vi "SaveConfigFile.vi"(0 "error in (no error)":errorcluster, 1 "IP":string caption="Robot IP Address", 2 "Licensee":string, 3 "Key":string, 4 "Username":string, 5 "Password":string) -> (20 "error out":errorcluster)   [LabVIEW 2011]
uses:
  <vilib>/Utility/config.llb/NI_LVConfig.lvlib
  <vilib>/Utility/config.llb/Write Key (String).vi
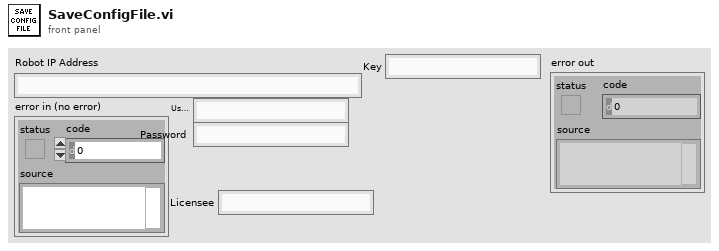
[diagram p1: front panel]
types:
  T1 = typedef "NI_LVConfig.lvlib/Config Data RefNum.ctl" = refnum<k1>
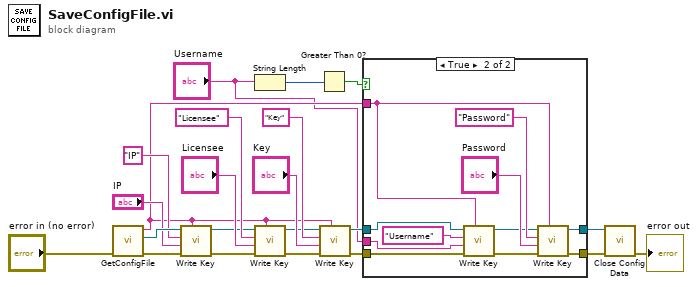
[diagram p0: block diagram]
diagram:
  n1 = call "GetConfigFile.vi"("error in (no error)"="error in (no error)") -> ("error out"=w21:errorcluster, "refnum"=w20:T1, "section"=w8:string)  [unwired: 8 in]
  n2 = call-poly <vilib>:"Write Key.vi"("section"=w8, "error in (no error)"=w21, "value"="IP", "key"="IP", "refnum"=w20) -> ("error out"=w9:errorcluster, "refnum out"=w10:T1)  [unwired: 4 in, 1 out]
  n3 = String Length(string="Username") -> (length=w2:i32)
  n4 = call-poly <vilib>:"Write Key.vi"("section"=w8, "error in (no error)"=w9, "value"="Licensee", "key"="Licensee", "refnum"=w10) -> ("error out"=w12:errorcluster, "refnum out"=w13:T1)  [unwired: 4 in, 1 out]
  n5 = Greater Than 0?(x=w2) -> (x > 0?=w1:bool)
  n6 = call-poly <vilib>:"Write Key.vi"("section"=w8, "error in (no error)"=w12, "value"="Key", "key"="Key", "refnum"=w13) -> ("error out"=w5:errorcluster, "refnum out"=w4:T1)  [unwired: 4 in, 1 out]
  n7 = case shown="True" w1 {
    tunnel: w8 -> [_ w32]
    tunnel: [w24 w30] -> w7
    tunnel: [w23 w29] -> w6
    tunnel: w5 -> [w23 w27]
    tunnel: w4 -> [w24 w26]
    tunnel: "Username" -> [_ w25]
    frame False {
    }
    frame True {
      n8 = call-poly <vilib>:"Write Key.vi"("section"=w32, "error in (no error)"=w27, "value"=w25, "key"="Username", "refnum"=w26) -> ("error out"=w28:errorcluster, "refnum out"=w31:T1)  [unwired: 4 in, 1 out]
      n9 = call-poly <vilib>:"Write Key.vi"("section"=w32, "error in (no error)"=w28, "value"="Password", "key"="Password", "refnum"=w31) -> ("error out"=w29:errorcluster, "refnum out"=w30:T1)  [unwired: 4 in, 1 out]
    }
  }
  n10 = call <vilib>:"Close Config Data.vi"("error in (no error)"=w6, "refnum"=w7) -> ("error out"=→"error out":errorcluster)  [unwired: 8 in, 1 out]
